vi "Aula dia 05.02.vi"() -> ()   [LabVIEW 2020]
uses:
  <vilib>/numeric/Random Number (Range) DBL.vi
panel:
  out "Potência Ativa  A 3":dbl[](graph)
  out "Tensão C":dbl[](array[numeric])
  out "Corrente C":dbl[](array[numeric])
  out "Potência Ativa A 3":dbl[](array[numeric])
  out "Potência Ativa A 2":dbl[](array[numeric])
  out "Corrente B":dbl[](array[numeric])
  out "Tensão B":dbl[](array[numeric])
  out "Potência Ativa  A 2":dbl[](graph)
  out "Potência Ativa A":dbl[](array[numeric])
  out "Corrente A":dbl[](array[numeric])
  out "Tensão A":dbl[](array[numeric])
  out "Fator de Potência":dbl
  in  "Limite Superior FP":dbl
  in  "Limite Inferior FP":dbl=100.0
  out "Potência Ativa  A":dbl[](graph)
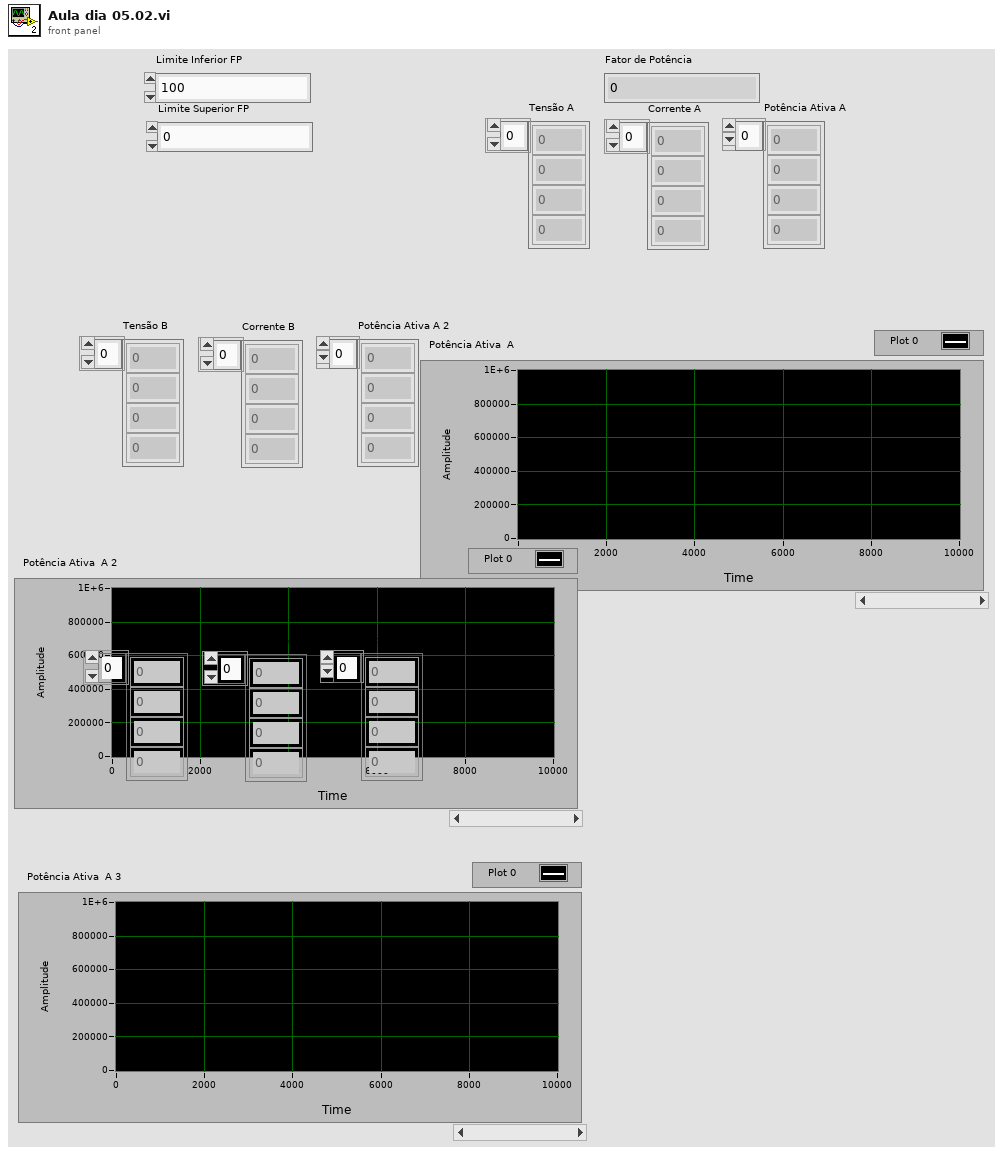
[diagram p1: front panel]
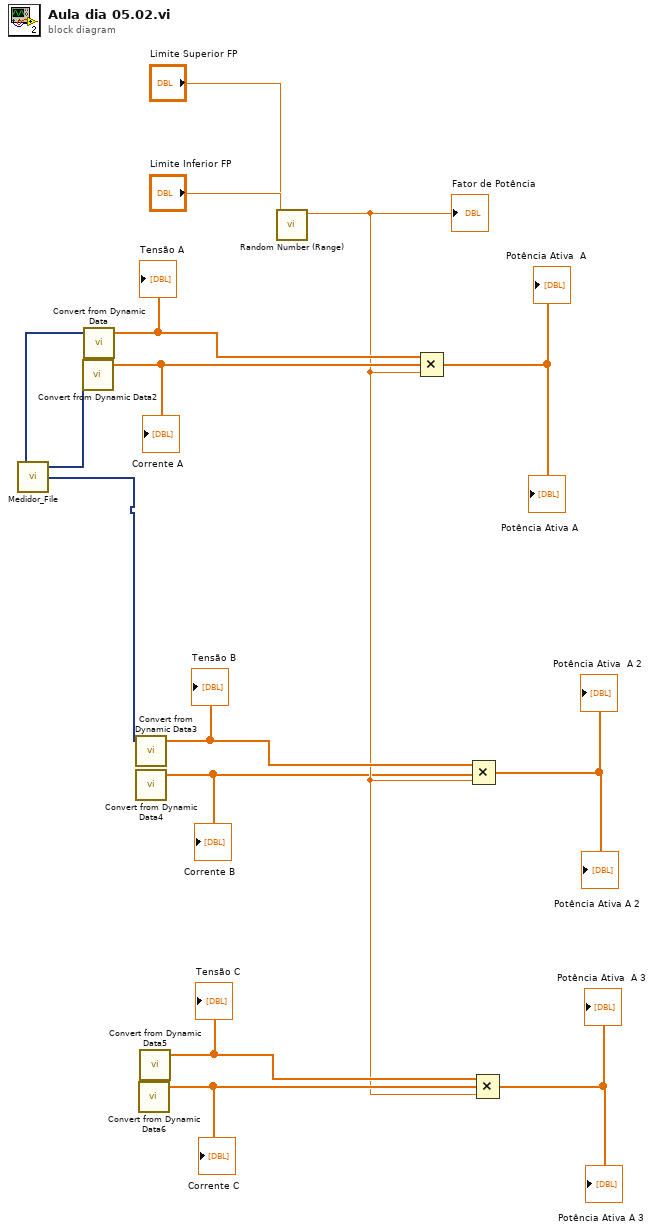
[diagram p0: block diagram]
diagram:
  n1 = call "Medidor_File.vi"() -> ("Corrente Fase B"=w1:dynamicdata, "Corrente Fase A"=w15:dynamicdata, "Tensão Fase A"=w14:dynamicdata)  [unwired: 4 out]
  n2 = call "Convert from Dynamic Data2"("Dynamic Data Type"=w15) -> ("Array"=w12:dbl[])  [unwired: 3 in]
  "Corrente A" <- w12
  n3 = call "Convert from Dynamic Data"("Dynamic Data Type"=w14) -> ("Array"=w13:dbl[])  [unwired: 3 in]
  "Tensão A" <- w13
  n4 = call "Convert from Dynamic Data3"("Dynamic Data Type"=w1) -> ("Array"=w7:dbl[])  [unwired: 3 in]
  "Tensão B" <- w7
  n5 = call "Convert from Dynamic Data4"() -> ("Array"=w2:dbl[])  [unwired: 4 in]
  "Corrente B" <- w2
  n6 = call "Convert from Dynamic Data6"() -> ("Array"=w4:dbl[])  [unwired: 4 in]
  "Corrente C" <- w4
  n7 = call "Convert from Dynamic Data5"() -> ("Array"=w6:dbl[])  [unwired: 4 in]
  "Tensão C" <- w6
  n8 = call-poly <vilib>:"Random Number (Range).vi"("lower bound (0)"="Limite Superior FP", "upper bound (100)"="Limite Inferior FP") -> ("number"=w3:dbl)  [unwired: 9 in]
  "Fator de Potência" <- w3
  n9 = Compound Arithmetic op=MULTIPLY(w13, w12, w3) -> (→"Potência Ativa  A" →"Potência Ativa A":dbl[])
  n10 = Compound Arithmetic op=MULTIPLY(w7, w2, w3) -> (→"Potência Ativa  A 2" →"Potência Ativa A 2":dbl[])
  n11 = Compound Arithmetic op=MULTIPLY(w6, w4, w3) -> (→"Potência Ativa  A 3" →"Potência Ativa A 3":dbl[])
